vi "kamerka_cofania.vi"() -> ()   [LabVIEW 2023]
doc: "Use this template to build a standard state machine design pattern. Each state executes code and determines which state to transition to. Contrast this design pattern with the User Interface Event Handler pattern, in which code executes in response to user actions. Contrast this design pattern also with the Queued Message Handler pattern, in which each message handling code can queue zero or more new messages.\nNote: This template does not contain the most recent programming guidelines recommended by National Instruments. For a complete, project-based implementation of the Standard State Machine pattern, use the Create Project dialog box instead of this template."
uses:
  <vilib>/userDefined/High Color/IMAQdx.ctl
  Downloads/wasilistan.ctl
  <vilib>/vision/Image Controls.llb/IMAQ Image.ctl
  <vilib>/Instr/_visa.llb/VISA Configure Serial Port (Instr).vi
  <vilib>/regexp/Match Regular Expression.xnode
  <vilib>/vision/driver/NI_Vision_Acquisition_Software.lvlib
panel:
  out "Image":T1(plugin-control)
  in  "Kamerka 2":T2
  out "error out 2":errorcluster
  in  "Arduino":refnum<visa-resource-name>
  in  "symulator odleglosci":dbl
  out "Serial Settings:Number of Bytes at Serial Port":u32
  in  "STOP":bool
  out "Odleglosc":dbl
  out "read buffer":string
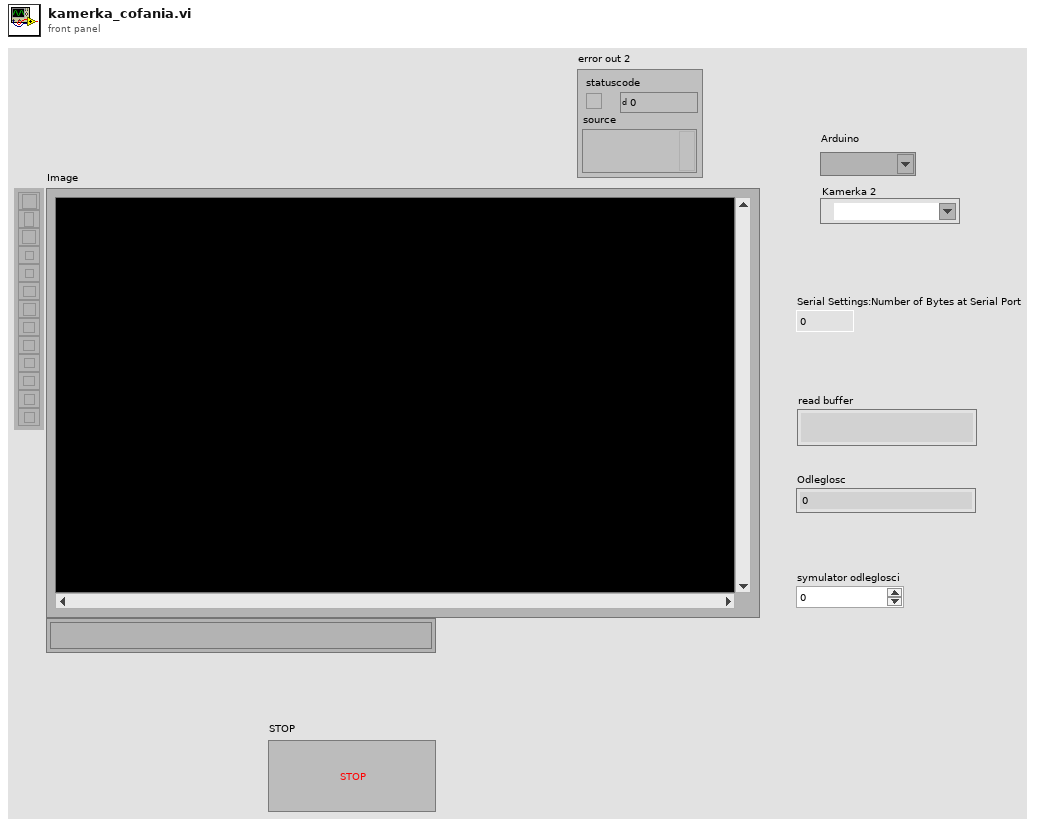
[diagram p1: front panel]
types:
  T1 = typedef "IMAQ Image.ctl" = refnum<image>
  T2 = typedef "IMAQdx.ctl" = refnum<k21>
  T3 = typedef "wasilistan.ctl" = enum16{"Initialize", "Czytaj", "Buzzer", "Kamera", "Stop"}
  T4 = typedef "Image Type" = u32
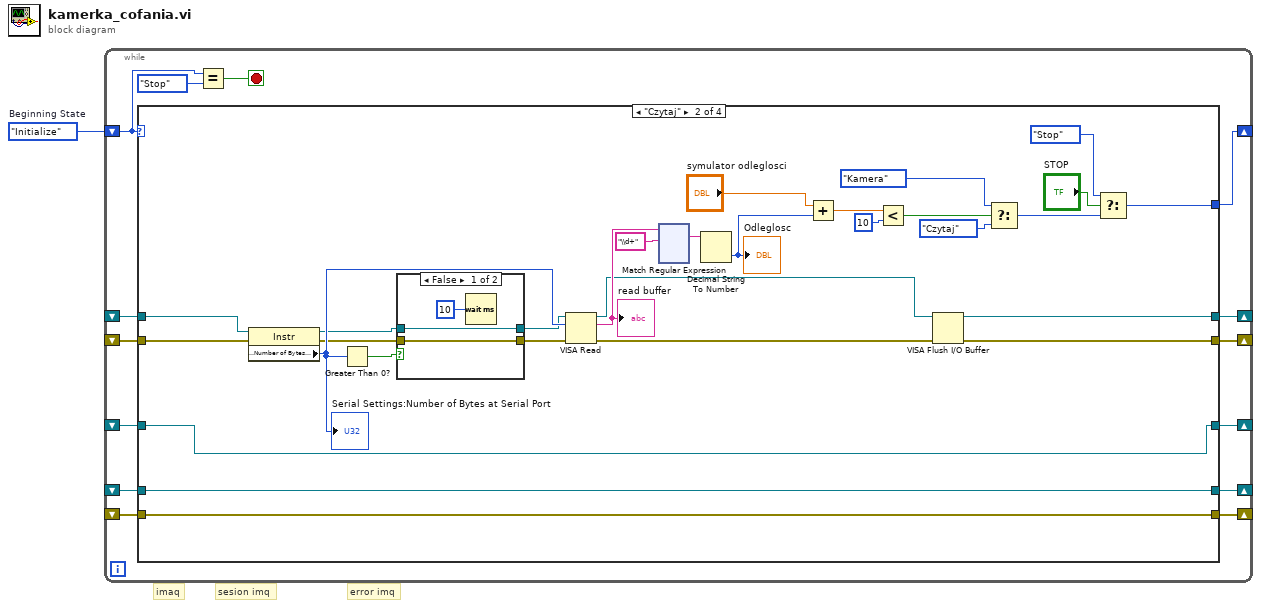
[diagram p0: block diagram]
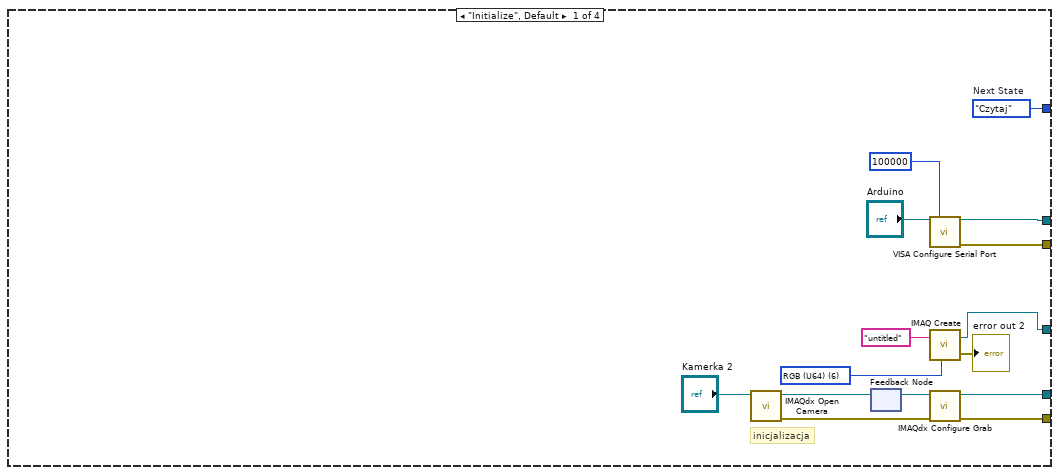
[diagram p2: hidden frame]
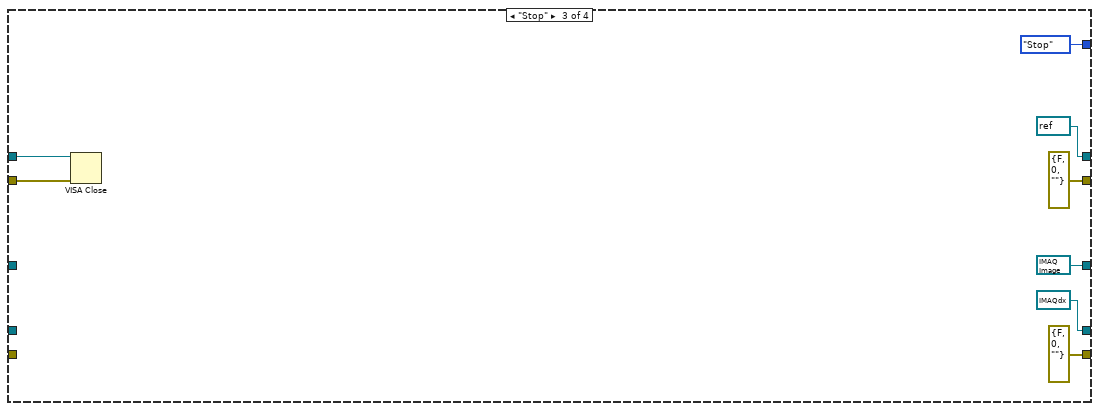
[diagram p4: hidden frame]
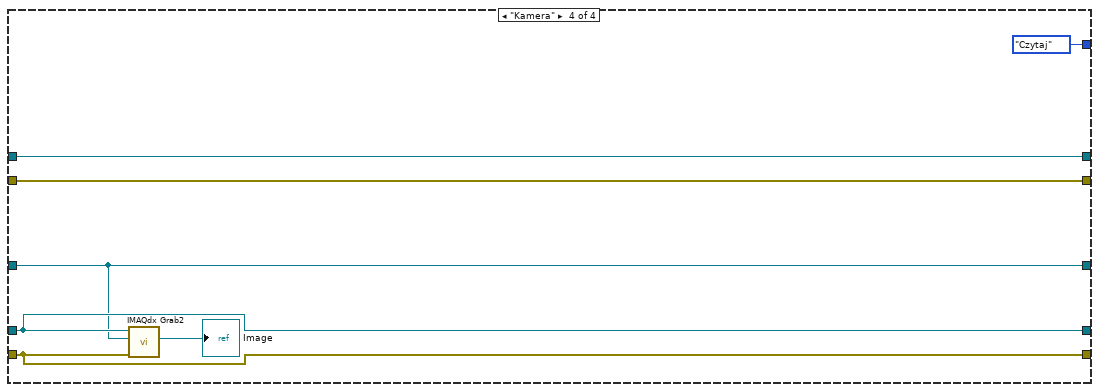
[diagram p5: hidden frame]
diagram:
  w1 = wasilistan."Initialize"  # Beginning State
  # "sesion imq"
  # "error imq"
  # "imaq"
  n1 = while {
    shift-right: [w13] -> _
    shift-left: w1 -> [w8]
    shift-right: [w12] -> _
    shift-left: _ -> [w10]
    shift-right: [w11] -> _
    shift-left: _ -> [w9]
    shift-right: [w7] -> _
    shift-left: _ -> [w2]
    shift-right: [w6] -> _
    shift-left: _ -> [w3]
    shift-right: [w5] -> _
    shift-left: _ -> [w4]
    stop <- w15 stop-if-true
    n2 = case shown="\"Czytaj\"" w8 {
      tunnel: [w30 w56 wasilistan."Stop" ("Next State") wasilistan."Czytaj"] -> w13
      tunnel: [w28 w42 refnum<visa-resource-name> refnum ("VISA resource name out") w191] -> w12
      tunnel: [w27 w43 errorcluster {"status"=FALSE, "code"=0, "source"=""} ("error constant") w190] -> w11
      tunnel: w10 -> [_ w34 w188 w191]
      tunnel: w9 -> [_ w33 w187 w190]
      tunnel: [w18 w35 T1 refnum ("New Image") w193] -> w7
      tunnel: [w17 w36 errorcluster {"status"=FALSE, "code"=0, "source"=""} ("error out") w192] -> w6
      tunnel: [w16 w37 T2 refnum ("Session Out") w194] -> w5
      tunnel: w4 -> [_ w37 _ w194]
      tunnel: w3 -> [_ w36 _ w192]
      tunnel: w2 -> [_ w35 _ w193]
      frame "Initialize", Default {
        w20 = T4 6 items=["Grayscale (U8)", "Grayscale (I16)", "Grayscale (SGL)", "Complex (CSG)", "RGB (U32)", "HSL (U32)", "RGB (U64)", "Grayscale (U16)"] ("Image Type")
        w30 = wasilistan."Czytaj"  # Next State
        # "inicjalizacja"
        n3 = call <vilib>:"IMAQdx Open Camera.vi"("Session In"="Kamerka 2") -> ("error out"=w23:errorcluster, "Session Out"=w25:T2)  [unwired: 9 in]
        n4 = feedback #1() -> (w24:T2)  [unwired: 1 in]
        n5 = feedback-in #1(w25) -> ()
        n6 = call-poly "VISA Configure Serial Port"("VISA resource name"="Arduino", "timeout (10sec)"=u32 100000) -> ("VISA resource name out"=w28:refnum<visa-resource-name>, "error out"=w27:errorcluster)  [unwired: 12 in]
        n7 = call "IMAQ Create"("Image Name"="untitled", "Image Type"=w20) -> ("New Image"=w18:T1, "error out"=→"error out 2":errorcluster)  [unwired: 3 in]
        n8 = call <vilib>:"IMAQdx Configure Grab.vi"("error in"=w23, "Session In"=w24) -> ("error out"=w17:errorcluster, "Session Out"=w16:T2)  [unwired: 8 in]
      }
      frame "Czytaj" {
        n9 = property class="Instr"(reference=w34, error in=w33) -> (reference out=w48:refnum<visa-resource-name>, error out=w46:errorcluster, "Serial Settings:Number of Bytes at Serial Port"=w50:u32)
        "Serial Settings:Number of Bytes at Serial Port" <- w50
        n10 = Greater Than 0?(x=w50) -> (x > 0?=w49:bool)
        n11 = case shown="False" w49 {
          tunnel: [w62 w64] -> w47
          tunnel: w48 -> [w62 w64]
          tunnel: w46 -> [w61 w63]
          tunnel: [w61 w63] -> w45
          frame False {
            n12 = Wait (ms)(milliseconds to wait=u32 10) -> ()  [unwired: 1 out]
          }
          frame True {
          }
        }
        n13 = VISA Read(VISA resource name=w47, byte count=w50, error in (no error)=w45) -> (VISA resource name out=w41:refnum<visa-resource-name>, read buffer=w44:string, error out=w40:errorcluster)  [unwired: 1 out]
        "read buffer" <- w44
        n14 = xnode "Match Regular Expression"("input string"=w44, "regular expression"="\\d+") -> ("whole match"=w58:string)  [unwired: 4 in, 4 out]
        n15 = Decimal String To Number(string=w58) -> (number=w51:i32)  [unwired: 2 in, 1 out]
        "Odleglosc" <- w51
        n16 = Add(x="symulator odleglosci", y=w51) -> (x+y=w38:dbl)
        n17 = Less?(x=w38, y=10) -> (x < y?=w32:bool)
        n18 = VISA Flush I/O Buffer(VISA resource name=w41, error in (no error)=w40) -> (VISA resource name out=w42:refnum<visa-resource-name>, error out=w43:errorcluster)  [unwired: 1 in]
        n19 = Select(t=wasilistan."Kamera", s=w32, f=wasilistan."Czytaj") -> (s? t:f=w54:T3)
        n20 = Select(t=wasilistan."Stop", s="STOP", f=w54) -> (s? t:f=w56:T3)
      }
      frame "Stop" {
        n21 = VISA Close(VISA resource name=w188, error in (no error)=w187) -> ()  [unwired: 1 out]
      }
      frame "Kamera" {
        n22 = call <vilib>:"IMAQdx Grab2.vi"("error in"=w192, "Image In"=w193, "Session In"=w194) -> ("Image Out"=→"Image":T1)  [unwired: 5 in, 3 out]
      }
    }
    n23 = Equal?(x=w8, y=wasilistan."Stop" ("States")) -> (x = y?=w15:bool)
  }
